vi "Write Category Name.vi"(8 "error in (no error)":errorcluster, 10 "Category Name":string, 11 "Config Plugin in":refnum<class "Config Plugin.lvclass">) -> (0 "error out":errorcluster, 3 "Config Plugin out":refnum<class "Config Plugin.lvclass">)   [LabVIEW 2016, in "Config Plugin.lvlib" / "Config Plugin.lvclass"]
uses:
  <userlib>/Common Components/Config Plugin/Config Plugin.lvclass
  <userlib>/Common Components/Config Plugin/Config Plugin.lvclass/Config Plugin.ctl
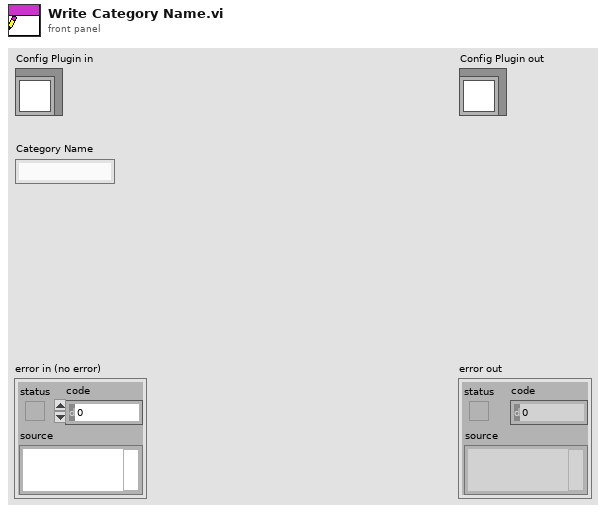
[diagram p1: front panel]
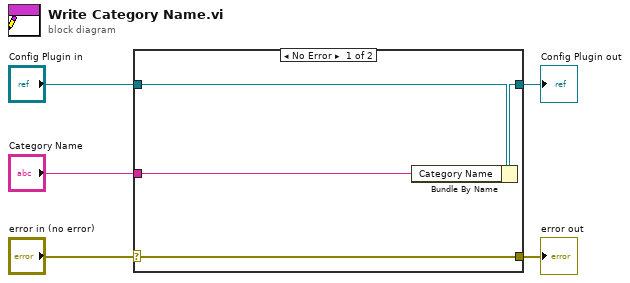
[diagram p0: block diagram]
diagram:
  n1 = case shown="No Error" "error in (no error)" {
    selector: "error in (no error)" -> [w9 w10]
    tunnel: [w9 w10] -> w4
    tunnel: [w7 w11] -> w2
    tunnel: "Config Plugin in" -> [w8 w11]
    tunnel: "Category Name" -> [w6 _]
    frame No Error {
      n2 = Bundle By Name(cluster=w8, "Category Name"=w6) -> (w7:refnum<class "Config Plugin.lvclass">)
    }
    frame Error {
    }
  }
  "error out" <- w4
  "Config Plugin out" <- w2
